vi "Check if Open or Locked.vi"(8 "error in (no error)":errorcluster, 11 "Standard VI Type in":refnum<class "Standard VI Type.lvclass">) -> (0 "error out":errorcluster, 3 "Openable?":bool)   [LabVIEW 2020, in "Peek Window.lvlib" / "Standard VI Type.lvclass"]
uses:
  Standard VI Type.lvclass
  Standard VI Type.lvclass/Standard VI Type.ctl
  f27b3d3e-214f-402c-a623-d144d9039078.vi
  Read VI Refnum.vi
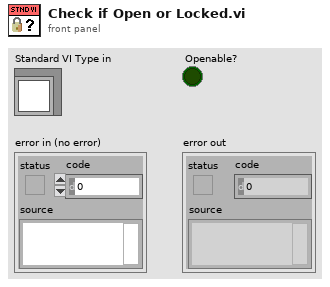
[diagram p1: front panel]
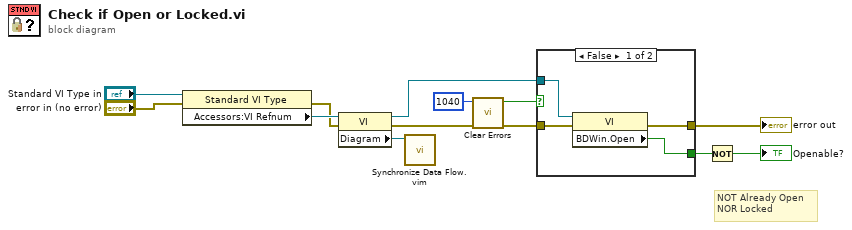
[diagram p0: block diagram]
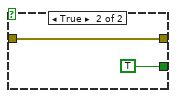
[diagram p2: hidden frame]
diagram:
  # "NOT Already Open\nNOR Locked"
  n1 = property class="Standard VI Type"(reference="Standard VI Type in", error in="error in (no error)") -> (error out=w6:errorcluster, "Accessors:VI Refnum"=w7:refnum<vi>)  [unwired: 1 out]
  n2 = property class="VI"(reference=w7, error in=w6) -> (reference out=w9:refnum<vi>, error out=w12:errorcluster, "Diagram"=w8:refnum<vi>)
  n3 = call "Synchronize Data Flow.vim"("input 1"=w8) -> ()  [unwired: 3 in, 4 out]
  n4 = call <vilib>:"Clear Errors.vi"("error in (no error)"=w12, "specific error code to clear (0: all)"=1040) -> ("error out"=w10:errorcluster, "specific error cleared?"=w11:bool)  [unwired: 4 in]
  n5 = case shown="False" w11 {
    tunnel: w10 -> [w17 w19]
    tunnel: [w16 w19] -> w3
    tunnel: [w14 TRUE ("Locked or Open?")] -> w2
    tunnel: w9 -> [w15 _]
    frame False {
      n6 = property class="VI"(reference=w15, error in=w17) -> (error out=w16:errorcluster, "BDWin.Open"=w14:bool)  [unwired: 1 out]
    }
    frame True {
    }
  }
  "error out" <- w3
  n7 = Not(x=w2) -> (.not. x?=→"Openable?":bool)
